vi "Joystick Gain.vi"(10 "input":dbl(slide) scale=-1.0..1.0, 11 "Sensitivity":dbl=1.0 format="%#_13g") -> (3 "output":dbl)   [LabVIEW 2019, in "Joysticks.lvlib" / "Joysticks.lvclass"]
doc: "This VI is used to scale the joystic to a cubic function, with the sensitivity changing how quick the stick responds"
uses:
  Joysticks.lvclass
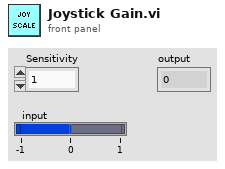
[diagram p1: front panel]
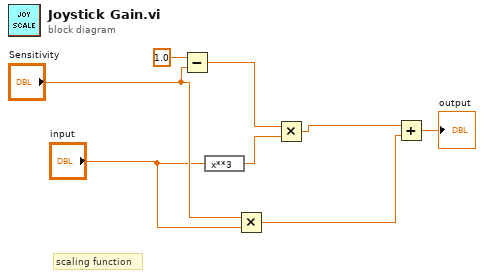
[diagram p0: block diagram]
diagram:
  # "scaling function"
  n1 = Subtract(x=1.0, y="Sensitivity") -> (x-y=w5:dbl)
  n2 = expression code="x**3"("input") -> (w1:dbl)
  n3 = Multiply(x="Sensitivity", y="input") -> (x*y=w8:dbl)
  n4 = Multiply(x=w5, y=w1) -> (x*y=w7:dbl)
  n5 = Add(x=w7, y=w8) -> (x+y=→"output":dbl)
